vi "ANOVA of synthetic fiber.vi"() -> ()   [LabVIEW 2023]
doc: "This example demonstrates how to use Analysis of Variance (ANOVA) to investigate the tensile strength of a synthetic fiber. The factor is the percent of cotton used in the blend of the materials to generate the fiber."
uses:
  <vilib>/Analysis/NI_AALPro.lvlib
  <vilib>/Analysis/NI_AALBase.lvlib
panel:
  in  "Reject":string="Reject"
  in  "Accept":string="Accept"
  in  "Does not affect fiber":string="The treatment (concentration of cotton) does not affect the result (strength of the fiber). "
  in  "Affects fiber":string="The treatment (concentration of cotton) affects the strength of the fiber."
  in  "Tab Control":T1(tab)
  out "variance":dbl[](array[numeric])
  in  "observations":dbl[][](array[numeric])=[[7.0, 7.0, 12.0, 15.0, 9.0, 10.0], [12.0, 17.0, 12.0, 18.0, 18.0, 17.0], [14.0, 18.0, 18.0, 19.0, 19.0, 18.0], [19.0, 25.0, 22.0, 19.0, 23.0, 23.0], [7.0, 10.0, 11.0, 15.0, 11.0, 12.0]]
  in  "tensile strength observations":dbl[](array[numeric])=[1.0, 2.0, 3.0, 4.0, 5.0, 6.0]
  in  "percentage of cotton (levels)":dbl[](array[numeric])=[15.0, 20.0, 25.0, 30.0, 35.0]
  out "total":dbl[](array[numeric])
  out "average":dbl[](array[numeric])
  out "number of repetitions":i32
  out "number of levels":i32
  out "Hypothesis of Ho":string
  out "Conclusion":string
  out "ratio of msa/mse (Fo)":dbl format="%0.4f"
  out "Mean Square Error (MSe)":dbl format="%0.4f"
  out "Sum of Square Factor (SSa)":dbl format="%0.4f"
  out "Mean Square Factor (MSa)":dbl format="%0.4f"
  out "Sum of Squares Error (SSe)":dbl format="%0.4f"
  out "Total Sum of Squares (SSt)":dbl format="%0.4f"
  out "degree of freedom":i32
  out "degree of freedom 2":i32
  out "degree of freedom 3":i32
  in  "Level of significance":dbl=0.01
  out "Calculated level of significance":dbl format="%#.6g"
  out "Scatter Plot":T2(graph)
  # "Overview: Demonstrates the use of the 1D ANOVA VI to investigate the tensile strength of a synthetic fiber.\nRequirements: LabVIEW Full Development System\nInstructions: \n1. Run the VI.\n2. Verify the parameters on the Problem Statement and Data Entry tabs.\n3. On the Analysis of Variance tab, verify the results of the analysis and the conclusion of the experiment.\n4. On the Scatter Plot tab, observe the Mean and Data values for each level."
  # "Statistical analysis:"
  # "Where:\nm : mean value\nt : treatment effect\ne : measurement error\ni : number of treatments\nj : number of measurements"
  # "Hypothesis:"
  # "Ho : t1 = t2 =t3 =...= ti= 0 against H1 : ti <> 0 for at least one i."
  # "The hypothesis Ho means the measurements are only affected by noise, while the hypothesis H1 means the measurements are affected at least one treatment or level."
  # "Experiment:"
  # "Obtain 5 measurements for each of the 5 concentration of cotton (levels)."
  # "Analysis:"
  # "Source of\nVariation"
  # "Sum of \nSquares"
  # "Degrees of \nFreedom"
  # "Mean Square"
  # "Fo"
  # "Between"
  # "Within"
  # "Total"
  # ">"
  # "?"
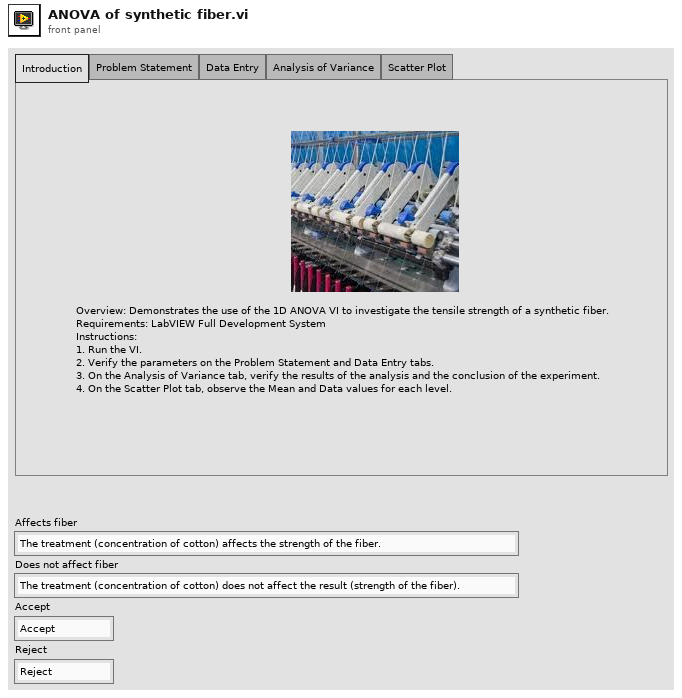
[diagram p1: front panel]
types:
  T1 = enum32{"Introduction", "Problem Statement", "Data Entry", "Analysis of Variance", "Scatter Plot"}
  T2 = cluster{"percentage of cotton (levels)":dbl[], "observations":dbl[]}[]
  T3 = cluster{"percentage of cotton (levels)":dbl[], dbl[]}
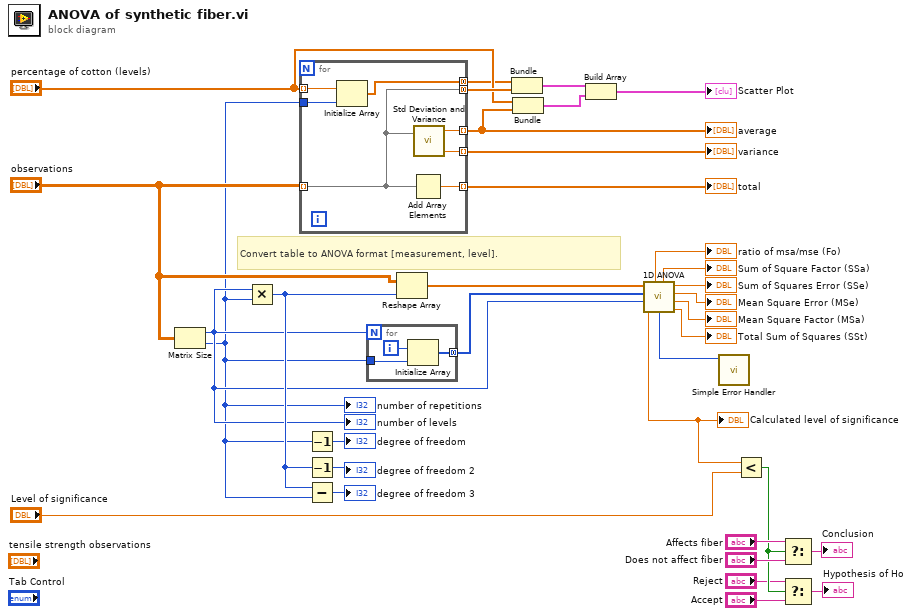
[diagram p0: block diagram]
diagram:
  # "Convert table to ANOVA format [measurement, level]."
  n1 = Matrix Size(0:"observations") -> (1:w14:i32, 2:w12:i32)
  "number of repetitions" <- w12
  "number of levels" <- w14
  n2 = Multiply(x=w14, y=w12) -> (x*y=w19:i32)
  n3 = for {
    tunnel: "observations" -> [w36] mode=indexing
    tunnel: [w41] -> w34 mode=indexing
    tunnel: [w35] -> w9 mode=indexing
    tunnel: [w40] -> w13 mode=indexing
    tunnel: "percentage of cotton (levels)" -> [w39] mode=indexing
    tunnel: [w38] -> w5 mode=concatenating
    tunnel: w12 -> [w37]
    tunnel: [w36] -> w11 mode=concatenating
    n4 = Initialize Array(w39, w37) -> (w38:dbl[])
    n5 = Add Array Elements(numeric array=w36) -> (sum=w41:dbl)
    n6 = call <vilib>:"Std Deviation and Variance.vi"("X"=w36) -> ("mean"=w35:dbl, "variance"=w40:dbl)  [unwired: 1 in, 1 out]
  }
  "total" <- w34
  "average" <- w9
  "variance" <- w13
  n7 = Decrement(x=w12) -> (x-1=→"degree of freedom":i32)
  n8 = Decrement(x=w19) -> (x-1=→"degree of freedom 2":i32)
  n9 = Subtract(x=w19, y=w12) -> (x-y=→"degree of freedom 3":i32)
  n10 = for {
    N: w14 -> [_]
    tunnel: w12 -> [w43]
    tunnel: [w42] -> w15 mode=concatenating
    i -> [w44]
    n11 = Initialize Array(w44, w43) -> (w42:i32[])
  }
  n12 = Reshape Array("observations", w19) -> (w30:dbl[])
  n13 = Bundle(w5, "observations"=w11) -> (w10:cluster{dbl[], "observations":dbl[]})  [unwired: 1 in]
  n14 = Bundle("percentage of cotton (levels)"="percentage of cotton (levels)", w9) -> (w8:T3)  [unwired: 1 in]
  n15 = Build Array(w10, w8) -> (→"Scatter Plot":T2)
  n16 = call <vilib>:"1D ANOVA.vi"("# of levels"=w14, "Index"=w15, "X"=w30) -> ("sig A"=w23:dbl, "error"=w32:i32, "tss"=→"Total Sum of Squares (SSt)":dbl, "msa"=→"Mean Square Factor (MSa)":dbl, "f"=→"ratio of msa/mse (Fo)":dbl, "mse"=→"Mean Square Error (MSe)":dbl, "ssa"=→"Sum of Square Factor (SSa)":dbl, "sse"=→"Sum of Squares Error (SSe)":dbl)
  "Calculated level of significance" <- w23
  n17 = call <vilib>:"Simple Error Handler.vi"("error code (no error:0)"=w32) -> ()  [unwired: 4 in, 5 out]
  n18 = Less?(x=w23, y="Level of significance") -> (x < y?=w4:bool)
  n19 = Select(t="Affects fiber", s=w4, f="Does not affect fiber") -> (s? t:f=→"Conclusion":string)
  n20 = Select(t="Reject", s=w4, f="Accept") -> (s? t:f=→"Hypothesis of Ho":string)
